vi "COMMAND_ResetController.vi"(8 "error in (no error)":errorcluster, 11 "StageDL090602SutterMP285 in":refnum<class "StageDL090602SutterMP285.lvclass">) -> (0 "error out":errorcluster, 3 "StageDL090602SutterMP285 out":refnum<class "StageDL090602SutterMP285.lvclass">)   [LabVIEW 2010, in "StageDL090602SutterMP285.lvclass"]
uses:
  StageDL090602SutterMP285.lvclass
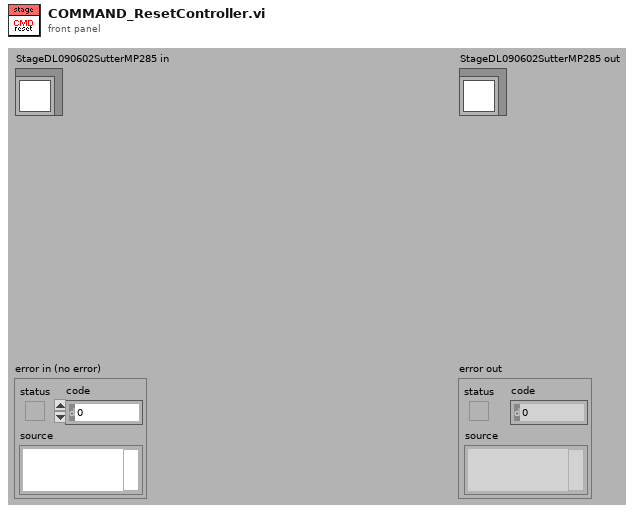
[diagram p1: front panel]
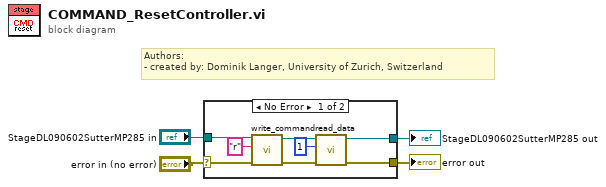
[diagram p0: block diagram]
diagram:
  # "Authors: \n- created by: Dominik Langer, University of Zurich, Switzerland"
  n1 = case shown="No Error" "error in (no error)" {
    selector: "error in (no error)" -> [w8 w14]
    tunnel: [w7 w14] -> w3
    tunnel: [w5 w13] -> w1
    tunnel: "StageDL090602SutterMP285 in" -> [w6 w13]
    frame No Error {
      n2 = call-dynamic "write_command.vi"("error in (no error)"=w8, "command (without terminating \"\\n\")"="r" ("command (without terminating \"\\n\")"), "DL090602SutterMP285Stage in"=w6) -> ("error out"=w9:errorcluster, "DL090602SutterMP285Stage out"=w11:refnum<class "StageDL090602SutterMP285.lvclass">)  [unwired: 7 in]
      n3 = call-dynamic "read_data.vi"("error in (no error)"=w9, "bytes to read"=u32 1, "DL090602SutterMP285Stage in"=w11) -> ("error out"=w7:errorcluster, "DL090602SutterMP285Stage out"=w5:refnum<class "StageDL090602SutterMP285.lvclass">)  [unwired: 6 in, 1 out]
    }
    frame Error {
    }
  }
  "error out" <- w3
  "StageDL090602SutterMP285 out" <- w1
